vi "PH_Periodic_Sequencer.ProcCases.vi"(0 "i ref in":refnum<vi>, 1 "selector":string, 2 "Data":T1, 3 "call cluster":T2={"Object"="", "Selector"="", "CallType"=enum."synchronous", "Async Object"="", "Async Selector"="", "Data Descriptor"="", "Data"=[], "Error #"=0, "Expire"=0}, 5 "error in (no error)":errorcluster) -> (14 "i ref out":refnum<vi>, 17 "answer cluster":T2={"Object"="", "Selector"="", "CallType"=enum."synchronous", "Async Object"="", "Async Selector"="", "Data Descriptor"="", "Data"=[], "Error #"=0, "Expire"=0}, 19 "error out":errorcluster)   [LabVIEW 2014, in "PH_Periodic_Sequencer.lvlib"]
doc: "This method is called by a process from within the default case in the event loop. The methods of a class that are linked to events will be called from THIS method. Add your code here."
uses:
  PH_Periodic_Sequencer.lvlib
  CS_Core/CSSystem/CoreDefs/CoreDefs.call_type.ctl
  CS_Core/BaseProcess/BaseProcess.descriptor string definition.ctl
  CS_Core/CSSystem/CoreDefs/CoreDefs.rawDataType.ctl
  PH_Basics/PH_StatusHandler/PH_StatusHandler.Status.ctl
  CS_Core/CSSystem/CoreLib/CoreLib.string 2 byte array.vi
  CS_Core/CSSystem/CoreLib/CoreLib.byte array 2 short.vi
  CS_Core/CSSystem/CoreLib/CoreLib.byte array 2 double.vi
  CS_Core/CSSystem/CoreLib/CoreLib.byte array 2 int.vi
  CS_Core/BaseProcess/BaseProcess.lvlib
  CS_Core/CAEObj/CAEObj.lvlib
  CS_Core/CSSystem/CoreLib/CoreLib.lvlib
  PH_Basics/PH_StatusHandler/PH_StatusHandler.lvlib
  PH_Sequencer/PH_Sequencer.lvlib
  CS_Core/CSSystem/CSSystemLib/CSSystemLib.lvlib
  PH_Basics/PH_Common/PH_Common.lvlib
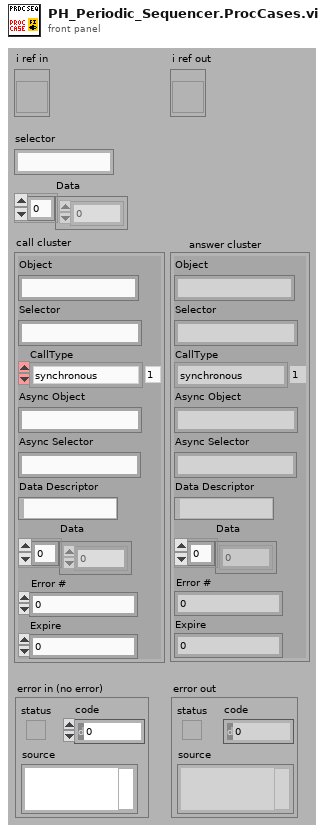
[diagram p1: front panel]
types:
  T1 = typedef "CoreDefs.rawDataType.ctl" = i8[]
  T2 = typedef "CoreDefs.call_type.ctl" = cluster{"Object":string, "Selector":string, "CallType":enum16{"simple", "synchronous", "asynchronous"}, "Async Object":string, "Async Selector":string, "Data Descriptor":T3, "Data":T1, "Error #":i32, "Expire":u32}
  T3 = typedef "BaseProcess.lvlib/BaseProcess.descriptor string definition.ctl" = string
  T4 = typedef "PH_Periodic_Sequencer.lvlib/PH_Periodic_Sequencer.i attribute.ctl" = cluster{"GUI Refs":cluster{"Main Off":refnum<vi>, "Start":refnum<vi>, "Ready":refnum<vi>, "Sequencer SM State":refnum<vi>, "Interval [sec]":refnum<vi>, "Wanted Shots":refnum<vi>, "Delivered Shots":refnum<vi>}, "PU Info":cluster{"Instancename":string, "State":T5, "linked":bool}[], "Sequencer":cluster{"Instancename":string, "linked?":bool, "R2S?":bool, "SM State":string}, "Run?":bool, "Interval [sec]":dbl, "PU State Refs":refnum<vi>[], "Wanted Shots":i32, "Delivered Shots":i32}
  T5 = typedef "PH_StatusHandler.lvlib/PH_StatusHandler.Status.ctl" = i16
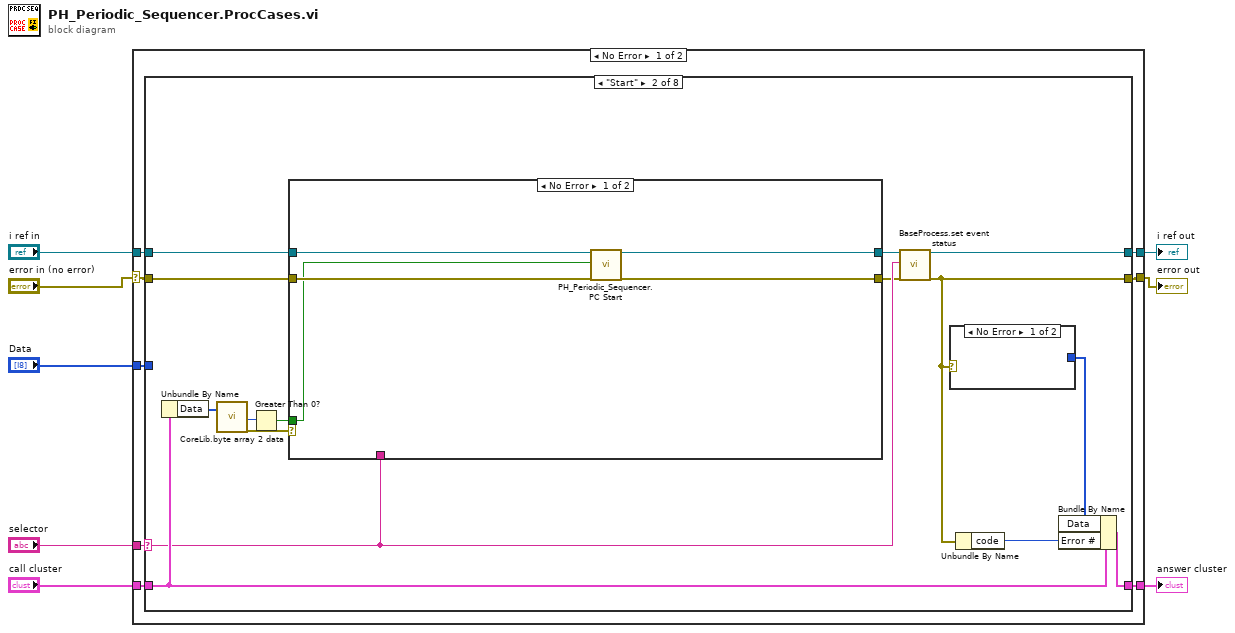
[diagram p0: block diagram]
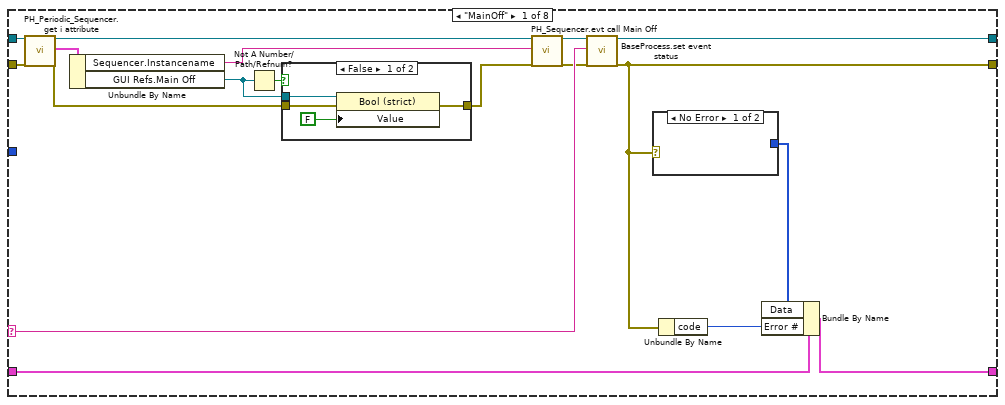
[diagram p2: hidden frame]
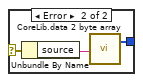
[diagram p3: hidden frame]
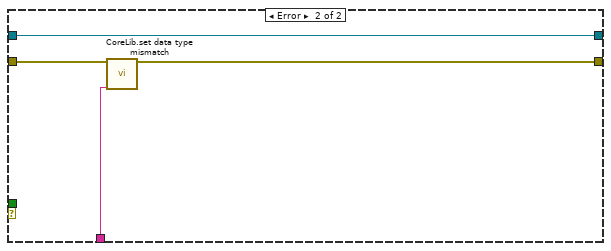
[diagram p5: hidden frame]
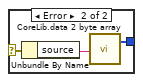
[diagram p6: hidden frame]
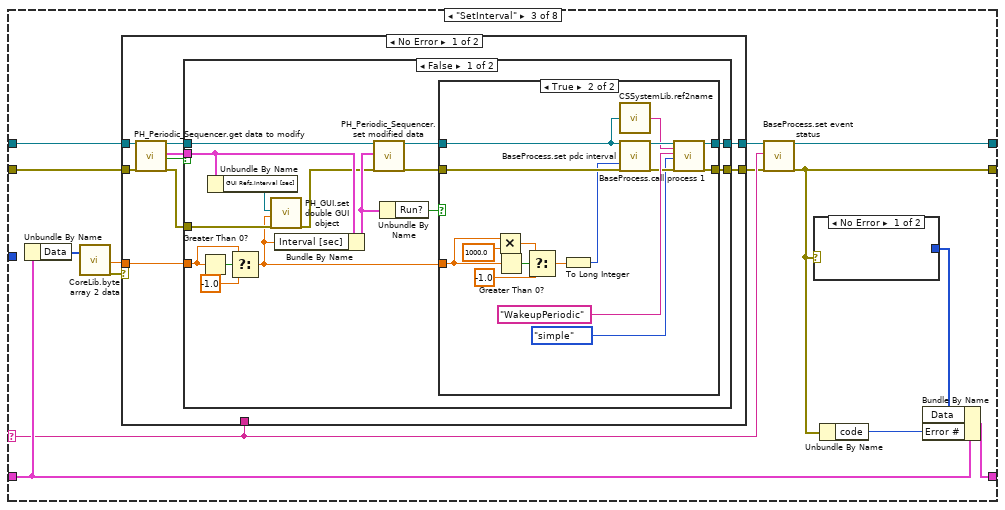
[diagram p7: hidden frame]
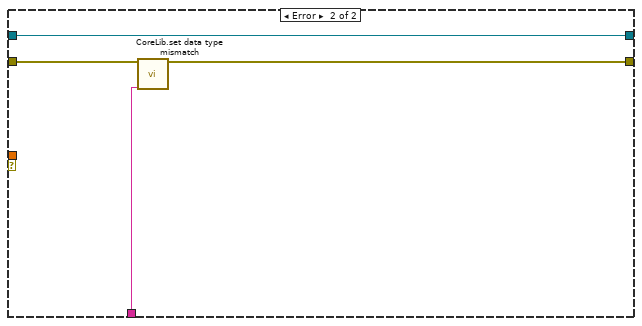
[diagram p10: hidden frame]
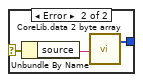
[diagram p11: hidden frame]
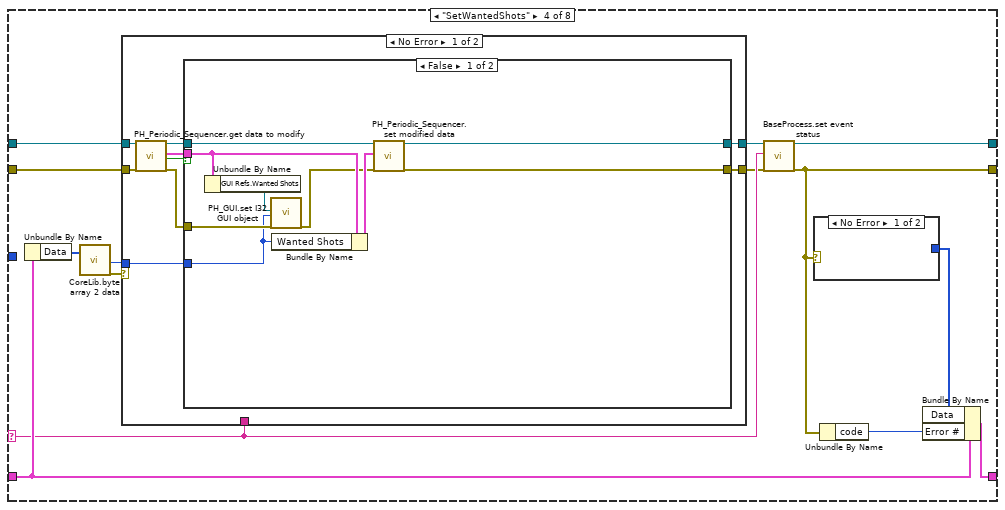
[diagram p12: hidden frame]
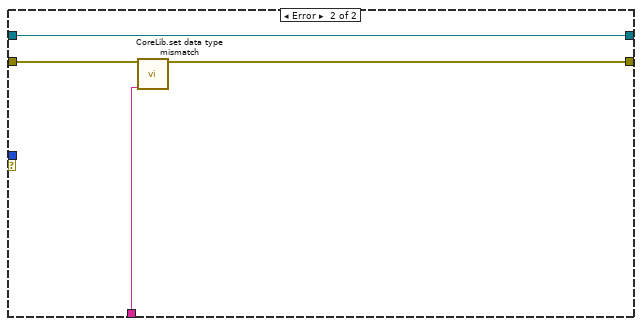
[diagram p14: hidden frame]
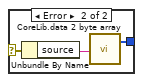
[diagram p15: hidden frame]
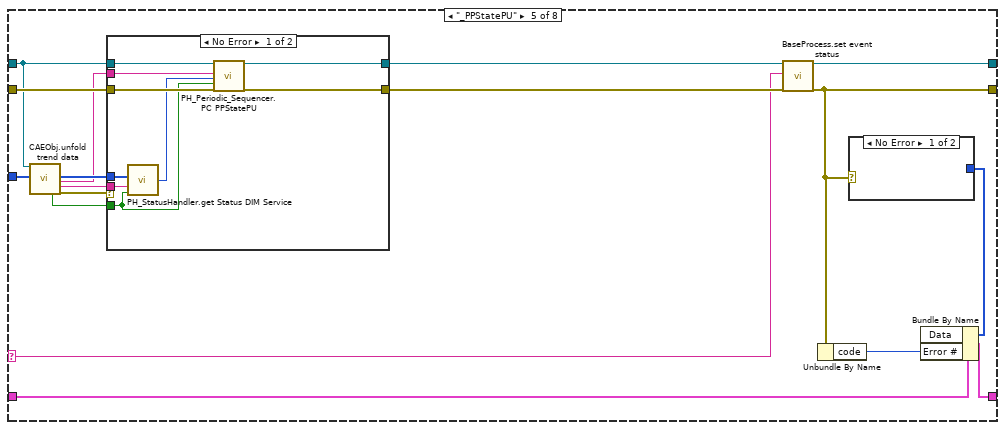
[diagram p16: hidden frame]
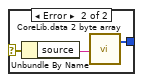
[diagram p17: hidden frame]
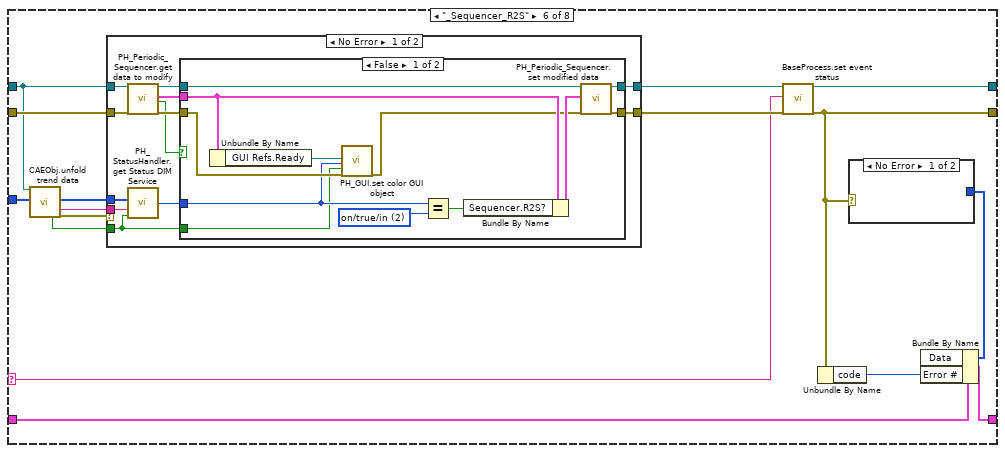
[diagram p19: hidden frame]
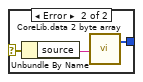
[diagram p20: hidden frame]
diagram:
  n1 = case shown="No Error" "error in (no error)" {
    selector: "error in (no error)" -> [w9 w295]
    tunnel: "selector" -> [w16 _]
    tunnel: [w15 w293] -> w7
    tunnel: "call cluster" -> [w14 w293]
    tunnel: "i ref in" -> [w13 w294]
    tunnel: [w12 w294] -> w4
    tunnel: [w11 w295] -> w3
    tunnel: "Data" -> [w10 _]
    frame No Error {
      n2 = case shown="\"Start\"" w16 {
        selector: w16 -> [w24 w48 w75 w140 w184 w214 w262 w287]
        tunnel: w13 -> [w30 w45 w72 w137 w181 w211 w259 w286]
        tunnel: [w26 w55 w81 w146 w187 w217 w265 w292] -> w12
        tunnel: w14 -> [w23 w50 w77 w142 w183 w213 w261 w288]
        tunnel: [w22 w53 w79 w144 w185 w215 w263 w289] -> w15
        tunnel: w9 -> [w29 w47 w74 w139 w192 w222 w270 w291]
        tunnel: [w25 w54 w80 w145 w186 w216 w264 w290] -> w11
        tunnel: w10 -> [_ _ _ _ w182 w212 w260 w285]
        frame "MainOff" {
          n3 = call "PH_Periodic_Sequencer.get i attribute.vi"("i ref in"=w30, "error in (no error)"=w29) -> ("i ref out"=w19:refnum<vi>, "i attribute"=w34:T4, "error out"=w33:errorcluster)  [unwired: 15 in]
          n4 = Unbundle By Name(w34) -> ("Sequencer.Instancename"=w17:string, "GUI Refs.Main Off"=w31:refnum<vi>)
          n5 = Not A Number/Path/Refnum?(number/path/refnum=w31) -> (NaN/Path/Refnum?=w32:bool)
          n6 = case shown="False" w32 {
            tunnel: w31 -> [w41 _]
            tunnel: w33 -> [w39 w42]
            tunnel: [w38 w42] -> w20
            frame False {
              n7 = property class="Bool (strict)"(reference=w41, error in=w39, "Value"=FALSE) -> (error out=w38:errorcluster)  [unwired: 1 out]
            }
            frame True {
            }
          }
          n8 = call "PH_Sequencer.evt call Main Off.vi"("i ref in"=w19, "Instance"=w17, "error in (no error)"=w20) -> ("i ref out"=w18:refnum<vi>, "error out"=w21:errorcluster)  [unwired: 15 in]
          n9 = call "BaseProcess.set event status.vi"("i ref in"=w18, "EventStatus"=w24, "error in (no error)"=w21) -> ("i ref out"=w26:refnum<vi>, "error out"=w25:errorcluster)  [unwired: 14 in, 1 out]
          n10 = case shown="No Error" w25 {
            selector: w25 -> [_ w37]
            tunnel: [_ w35] -> w27
            frame No Error {
            }
            frame Error {
              n11 = Unbundle By Name(w37) -> ("source"=w36:string)
              n12 = call-poly "CoreLib.data 2 byte array.vi"("string"=w36) -> ("byteArray out"=w35:T1)  [unwired: 18 in]
            }
          }
          n13 = Unbundle By Name(w25) -> ("code"=w28:i32)
          n14 = Bundle By Name(cluster=w23, "Data"=w27, "Error #"=w28) -> (w22:T2)
        }
        frame "Start" {
          n15 = Unbundle By Name(w50) -> ("Data"=w52:T1)
          n16 = call-poly "CoreLib.byte array 2 data.vi"("byteArray"=w52) -> ("i16"=w51:i16, "error out"=w49:errorcluster)  [unwired: 16 in, 1 out]
          n17 = Greater Than 0?(x=w51) -> (x > 0?=w43:bool)
          n18 = case shown="No Error" w49 {
            tunnel: w48 -> [_ w66]
            tunnel: w47 -> [w61 w65]
            tunnel: [w58 w64] -> w46
            tunnel: w45 -> [w62 w63]
            tunnel: [w59 w63] -> w44
            tunnel: w43 -> [w60 _]
            frame No Error {
              n19 = call "PH_Periodic_Sequencer.PC Start.vi"("i ref in"=w62, "Run?"=w60, "error IO"=w61) -> ("i ref out"=w59:refnum<vi>, "error out"=w58:errorcluster)  [unwired: 15 in]
            }
            frame Error {
              n20 = call "CoreLib.set data type mismatch.vi"("error in (no error)"=w65, "error source"=w66) -> ("error out"=w64:errorcluster)  [unwired: 17 in]
            }
          }
          n21 = call "BaseProcess.set event status.vi"("i ref in"=w44, "EventStatus"=w48, "error in (no error)"=w46) -> ("i ref out"=w55:refnum<vi>, "error out"=w54:errorcluster)  [unwired: 14 in, 1 out]
          n22 = case shown="No Error" w54 {
            selector: w54 -> [_ w69]
            tunnel: [_ w67] -> w56
            frame No Error {
            }
            frame Error {
              n23 = Unbundle By Name(w69) -> ("source"=w68:string)
              n24 = call-poly "CoreLib.data 2 byte array.vi"("string"=w68) -> ("byteArray out"=w67:T1)  [unwired: 18 in]
            }
          }
          n25 = Unbundle By Name(w54) -> ("code"=w57:i32)
          n26 = Bundle By Name(cluster=w50, "Data"=w56, "Error #"=w57) -> (w53:T2)
        }
        frame "SetInterval" {
          n27 = Unbundle By Name(w77) -> ("Data"=w78:T1)
          n28 = call-poly "CoreLib.byte array 2 data.vi"("byteArray"=w78) -> ("d64"=w70:dbl, "error out"=w76:errorcluster)  [unwired: 16 in, 1 out]
          n29 = case shown="No Error" w76 {
            tunnel: w75 -> [_ w131]
            tunnel: w74 -> [w92 w130]
            tunnel: [w87 w129] -> w73
            tunnel: w72 -> [w91 w128]
            tunnel: [w89 w128] -> w71
            tunnel: w70 -> [w84 _]
            frame No Error {
              n30 = call "PH_Periodic_Sequencer.get data to modify.vi"("i ref in"=w91, "error in (no error)"=w92) -> ("i ref out"=w90:refnum<vi>, "i attribute"=w85:T4, "timed out"=w86:bool, "error out"=w88:errorcluster)  [unwired: 14 in]
              n31 = case shown="False" w86 {
                tunnel: w90 -> [w107 w127]
                tunnel: [w105 w127] -> w89
                tunnel: w88 -> [w96 w126]
                tunnel: [w103 w126] -> w87
                tunnel: w85 -> [w98 _]
                tunnel: w84 -> [w99 _]
                frame False {
                  n32 = Greater Than 0?(x=w99) -> (x > 0?=w101:bool)
                  n33 = Unbundle By Name(w98) -> ("GUI Refs.Interval [sec]"=w97:refnum<vi>)
                  n34 = Select(t=w99, s=w101, f=-1.0) -> (s? t:f=w93:dbl)
                  n35 = call "PH_GUI.set double GUI object.vi"("GUI object Ref"=w97, "value"=w93, "error in (no error)"=w96) -> ("error out"=w95:errorcluster)  [unwired: 16 in]
                  n36 = Bundle By Name(cluster=w98, "Interval [sec]"=w93) -> (w102:T4)
                  n37 = call "PH_Periodic_Sequencer.set modified data.vi"("i ref in"=w107, "i attribute"=w102, "error in (no error)"=w95) -> ("i ref out"=w106:refnum<vi>, "error out"=w104:errorcluster)  [unwired: 15 in]
                  n38 = Unbundle By Name(w102) -> ("Run?"=w94:bool)
                  n39 = case shown="True" w94 {
                    tunnel: w106 -> [w109 w120]
                    tunnel: [w109 w119] -> w105
                    tunnel: w104 -> [w108 w118]
                    tunnel: [w108 w117] -> w103
                    tunnel: w93 -> [_ w111]
                    frame False {
                    }
                    frame True {
                      n40 = Multiply(x=w111, y=1000.0) -> (x*y=w113:dbl)
                      n41 = Greater Than 0?(x=w111) -> (x > 0?=w115:bool)
                      n42 = Select(t=w113, s=w115, f=-1.0) -> (s? t:f=w112:dbl)
                      n43 = To Long Integer(number=w112) -> (32bit integer=w110:i32)
                      n44 = call "CSSystemLib.ref2name.vi"("obj refnum"=w120) -> ("name"=w123:string)
                      n45 = call "BaseProcess.set pdc interval.vi"("i ref in"=w120, "PeriodicInterval [ms]"=w110, "error in (no error)"=w118) -> ("i ref out"=w125:refnum<vi>, "error out"=w122:errorcluster)  [unwired: 14 in, 1 out]
                      n46 = call "BaseProcess.call process 1.vi"("i ref in"=w125, "Object"=w123, "Selector"="WakeupPeriodic", "CallType"=enum16{"simple", "synchronous", "asynchronous"}."simple", "error in (no error)"=w122) -> ("i ref out"=w119:refnum<vi>, "error out"=w117:errorcluster)  [unwired: 12 in, 1 out]
                    }
                  }
                }
                frame True {
                }
              }
            }
            frame Error {
              n47 = call "CoreLib.set data type mismatch.vi"("error in (no error)"=w130, "error source"=w131) -> ("error out"=w129:errorcluster)  [unwired: 17 in]
            }
          }
          n48 = call "BaseProcess.set event status.vi"("i ref in"=w71, "EventStatus"=w75, "error in (no error)"=w73) -> ("i ref out"=w81:refnum<vi>, "error out"=w80:errorcluster)  [unwired: 14 in, 1 out]
          n49 = case shown="No Error" w80 {
            selector: w80 -> [_ w134]
            tunnel: [_ w132] -> w82
            frame No Error {
            }
            frame Error {
              n50 = Unbundle By Name(w134) -> ("source"=w133:string)
              n51 = call-poly "CoreLib.data 2 byte array.vi"("string"=w133) -> ("byteArray out"=w132:T1)  [unwired: 18 in]
            }
          }
          n52 = Unbundle By Name(w80) -> ("code"=w83:i32)
          n53 = Bundle By Name(cluster=w77, "Data"=w82, "Error #"=w83) -> (w79:T2)
        }
        frame "SetWantedShots" {
          n54 = Unbundle By Name(w142) -> ("Data"=w143:T1)
          n55 = call-poly "CoreLib.byte array 2 data.vi"("byteArray"=w143) -> ("i32"=w135:i32, "error out"=w141:errorcluster)  [unwired: 16 in, 1 out]
          n56 = case shown="No Error" w141 {
            tunnel: w140 -> [_ w172]
            tunnel: w139 -> [w157 w171]
            tunnel: [w152 w170] -> w138
            tunnel: w137 -> [w156 w169]
            tunnel: [w154 w169] -> w136
            tunnel: w135 -> [w149 _]
            frame No Error {
              n57 = call "PH_Periodic_Sequencer.get data to modify.vi"("i ref in"=w156, "error in (no error)"=w157) -> ("i ref out"=w155:refnum<vi>, "i attribute"=w150:T4, "timed out"=w151:bool, "error out"=w153:errorcluster)  [unwired: 14 in]
              n58 = case shown="False" w151 {
                tunnel: w155 -> [w166 w168]
                tunnel: [w159 w168] -> w154
                tunnel: w153 -> [w162 w167]
                tunnel: [w158 w167] -> w152
                tunnel: w150 -> [w164 _]
                tunnel: w149 -> [w160 _]
                frame False {
                  n59 = Unbundle By Name(w164) -> ("GUI Refs.Wanted Shots"=w163:refnum<vi>)
                  n60 = call "PH_GUI.set I32 GUI object.vi"("I32 GUI Ref"=w163, "value"=w160, "error in (no error)"=w162) -> ("error out"=w161:errorcluster)  [unwired: 16 in]
                  n61 = Bundle By Name(cluster=w164, "Wanted Shots"=w160) -> (w165:T4)
                  n62 = call "PH_Periodic_Sequencer.set modified data.vi"("i ref in"=w166, "i attribute"=w165, "error in (no error)"=w161) -> ("i ref out"=w159:refnum<vi>, "error out"=w158:errorcluster)  [unwired: 15 in]
                }
                frame True {
                }
              }
            }
            frame Error {
              n63 = call "CoreLib.set data type mismatch.vi"("error in (no error)"=w171, "error source"=w172) -> ("error out"=w170:errorcluster)  [unwired: 17 in]
            }
          }
          n64 = call "BaseProcess.set event status.vi"("i ref in"=w136, "EventStatus"=w140, "error in (no error)"=w138) -> ("i ref out"=w146:refnum<vi>, "error out"=w145:errorcluster)  [unwired: 14 in, 1 out]
          n65 = case shown="No Error" w145 {
            selector: w145 -> [_ w175]
            tunnel: [_ w173] -> w147
            frame No Error {
            }
            frame Error {
              n66 = Unbundle By Name(w175) -> ("source"=w174:string)
              n67 = call-poly "CoreLib.data 2 byte array.vi"("string"=w174) -> ("byteArray out"=w173:T1)  [unwired: 18 in]
            }
          }
          n68 = Unbundle By Name(w145) -> ("code"=w148:i32)
          n69 = Bundle By Name(cluster=w142, "Data"=w147, "Error #"=w148) -> (w144:T2)
        }
        frame "_PPStatePU" {
          n70 = call "CAEObj.unfold trend data.vi"("i ref in"=w181, "raw trend data"=w182) -> ("no link"=w179:bool, "data"=w178:i8[], "serviceName"=w177:string, "typeDescriptor"=w176:string, "error out"=w180:errorcluster)  [unwired: 9 in, 4 out]
          n71 = case shown="No Error" w180 {
            tunnel: [w199 w206] -> w188
            tunnel: w181 -> [w200 w206]
            tunnel: w192 -> [w202 w205]
            tunnel: [w201 w205] -> w189
            tunnel: w179 -> [w196 _]
            tunnel: w178 -> [w204 _]
            tunnel: w177 -> [w198 _]
            tunnel: w176 -> [w203 _]
            frame No Error {
              n72 = call "PH_StatusHandler.get Status DIM Service.vi"("no link"=w196, "typeDescriptor"=w203, "data"=w204) -> ("Status"=w197:T5)  [unwired: 1 in]
              n73 = call "PH_Periodic_Sequencer.PC PPStatePU.vi"("i ref in"=w200, "Service Name"=w198, "State"=w197, "not linked?"=w196, "error in (no error)"=w202) -> ("i ref out"=w199:refnum<vi>, "error out"=w201:errorcluster)  [unwired: 13 in]
            }
            frame Error {
            }
          }
          n74 = call "BaseProcess.set event status.vi"("i ref in"=w188, "EventStatus"=w184, "error in (no error)"=w189) -> ("i ref out"=w187:refnum<vi>, "error out"=w186:errorcluster)  [unwired: 14 in, 1 out]
          n75 = Unbundle By Name(w186) -> ("code"=w191:i32)
          n76 = case shown="No Error" w186 {
            selector: w186 -> [_ w195]
            tunnel: [_ w193] -> w190
            frame No Error {
            }
            frame Error {
              n77 = Unbundle By Name(w195) -> ("source"=w194:string)
              n78 = call-poly "CoreLib.data 2 byte array.vi"("string"=w194) -> ("byteArray out"=w193:T1)  [unwired: 18 in]
            }
          }
          n79 = Bundle By Name(cluster=w183, "Data"=w190, "Error #"=w191) -> (w185:T2)
        }
        frame "_Sequencer_R2S" {
          n80 = call "CAEObj.unfold trend data.vi"("i ref in"=w211, "raw trend data"=w212) -> ("no link"=w209:bool, "data"=w208:i8[], "typeDescriptor"=w207:string, "error out"=w210:errorcluster)  [unwired: 9 in, 5 out]
          n81 = case shown="No Error" w210 {
            tunnel: [w232 w253] -> w218
            tunnel: w211 -> [w234 w253]
            tunnel: w222 -> [w235 w252]
            tunnel: [w230 w252] -> w219
            tunnel: w209 -> [w226 _]
            tunnel: w208 -> [w237 _]
            tunnel: w207 -> [w236 _]
            frame No Error {
              n82 = call "PH_Periodic_Sequencer.get data to modify.vi"("i ref in"=w234, "error in (no error)"=w235) -> ("i ref out"=w233:refnum<vi>, "i attribute"=w228:T4, "timed out"=w229:bool, "error out"=w231:errorcluster)  [unwired: 14 in]
              n83 = call "PH_StatusHandler.get Status DIM Service.vi"("no link"=w226, "typeDescriptor"=w236, "data"=w237) -> ("Status"=w227:T5)  [unwired: 1 in]
              n84 = case shown="False" w229 {
                tunnel: w233 -> [w249 w251]
                tunnel: [w248 w251] -> w232
                tunnel: w231 -> [w242 w250]
                tunnel: [w247 w250] -> w230
                tunnel: w228 -> [w243 _]
                tunnel: w227 -> [w239 _]
                tunnel: w226 -> [w238 _]
                frame False {
                  w245 = T5 2 items=["no info", "off/false/out", "on/true/in", "Failure", "Alarm", "Status 1", "Status 2", "Status 3"] ("y")
                  n85 = Unbundle By Name(w243) -> ("GUI Refs.Ready"=w240:refnum<vi>)
                  n86 = call "PH_GUI.set color GUI object.vi"("GUI object Ref"=w240, "State"=w239, "Blinking? (false)"=w238, "error in (no error)"=w242) -> ("error out"=w241:errorcluster)  [unwired: 15 in]
                  n87 = Equal?(x=w239, y=w245) -> (x = y?=w244:bool)
                  n88 = Bundle By Name(cluster=w243, "Sequencer.R2S?"=w244) -> (w246:T4)
                  n89 = call "PH_Periodic_Sequencer.set modified data.vi"("i ref in"=w249, "i attribute"=w246, "error in (no error)"=w241) -> ("i ref out"=w248:refnum<vi>, "error out"=w247:errorcluster)  [unwired: 15 in]
                }
                frame True {
                }
              }
            }
            frame Error {
            }
          }
          n90 = call "BaseProcess.set event status.vi"("i ref in"=w218, "EventStatus"=w214, "error in (no error)"=w219) -> ("i ref out"=w217:refnum<vi>, "error out"=w216:errorcluster)  [unwired: 14 in, 1 out]
          n91 = Unbundle By Name(w216) -> ("code"=w221:i32)
          n92 = case shown="No Error" w216 {
            selector: w216 -> [_ w225]
            tunnel: [_ w223] -> w220
            frame No Error {
            }
            frame Error {
              n93 = Unbundle By Name(w225) -> ("source"=w224:string)
              n94 = call-poly "CoreLib.data 2 byte array.vi"("string"=w224) -> ("byteArray out"=w223:T1)  [unwired: 18 in]
            }
          }
          n95 = Bundle By Name(cluster=w213, "Data"=w220, "Error #"=w221) -> (w215:T2)
        }
        frame "_Sequencer_SM_State" {
          n96 = call "CAEObj.unfold trend data.vi"("i ref in"=w259, "raw trend data"=w260) -> ("quality"=w254:i32, "no link"=w257:bool, "data"=w256:i8[], "typeDescriptor"=w255:string, "error out"=w258:errorcluster)  [unwired: 9 in, 4 out]
          n97 = case shown="No Error" w258 {
            tunnel: [w279 w284] -> w266
            tunnel: w259 -> [w280 w284]
            tunnel: w270 -> [w282 w283]
            tunnel: [w281 w283] -> w267
            tunnel: w257 -> [w278 _]
            tunnel: w256 -> [w277 _]
            tunnel: w255 -> [w276 _]
            tunnel: w254 -> [w275 _]
            frame No Error {
              n98 = call "PH_DIM.get String.vi"("no link"=w278, "typeDescriptor"=w276, "data"=w277, "quality"=w275) -> ("Output String"=w274:string)
              n99 = call "PH_Periodic_Sequencer.PC StateSeqSM.vi"("i ref in"=w280, "SM State"=w274, "not linked?"=w278, "error in (no error)"=w282) -> ("i ref out"=w279:refnum<vi>, "error out"=w281:errorcluster)  [unwired: 14 in]
            }
            frame Error {
            }
          }
          n100 = call "BaseProcess.set event status.vi"("i ref in"=w266, "EventStatus"=w262, "error in (no error)"=w267) -> ("i ref out"=w265:refnum<vi>, "error out"=w264:errorcluster)  [unwired: 14 in, 1 out]
          n101 = Unbundle By Name(w264) -> ("code"=w269:i32)
          n102 = case shown="No Error" w264 {
            selector: w264 -> [_ w273]
            tunnel: [_ w271] -> w268
            frame No Error {
            }
            frame Error {
              n103 = Unbundle By Name(w273) -> ("source"=w272:string)
              n104 = call-poly "CoreLib.data 2 byte array.vi"("string"=w272) -> ("byteArray out"=w271:T1)  [unwired: 18 in]
            }
          }
          n105 = Bundle By Name(cluster=w261, "Data"=w268, "Error #"=w269) -> (w263:T2)
        }
        frame Default {
          # "In the default case, always call the ProcCase method of the parent class"
          n106 = call "BaseProcess.ProcCases.vi"("i ref in"=w286, "selector"=w287, "Data"=w285, "call cluster"=w288, "error in (no error)"=w291) -> ("i ref out"=w292:refnum<vi>, "answer cluster"=w289:T2, "error out"=w290:errorcluster)  [unwired: 12 in]
        }
      }
    }
    frame Error {
    }
  }
  "answer cluster" <- w7
  "i ref out" <- w4
  "error out" <- w3
